vi "From JSON Text (I32).vi"(7 "Default Value":i32, 9 "error in":errorcluster, 10 "Offset":i32, 11 "JSON":string) -> (1 "error out":errorcluster, 3 "Value":i32)   [LabVIEW 2021, in "json.facade.lvlib"]
doc: "Convert JSON to the LabVIEW Data Type entered."
uses:
  jsontext/LVClass Serializer/JSONtext LVClass Serializer.lvclass
  json.facade.lvlib
  jsontext/JSONtext.lvlib
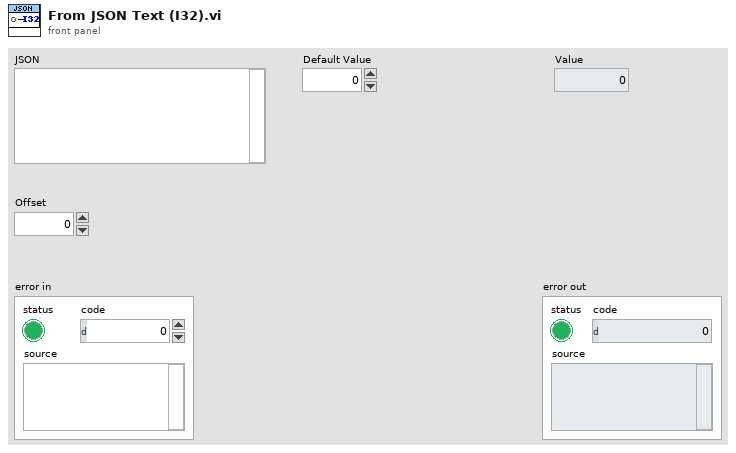
[diagram p1: front panel]
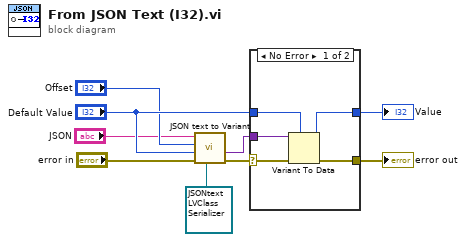
[diagram p0: block diagram]
diagram:
  n1 = call "JSON text to Variant.vi"("LVClass Serializer"=refnum<class "JSONtext LVClass Serializer.lvclass"> refnum, "error in (no error)"="error in", "Data Type"="Default Value", "Offset"="Offset", "JSON"="JSON") -> ("error out"=w2:errorcluster, "Variant out"=w3:variant)  [unwired: 5 in]
  n2 = case shown="No Error" w2 {
    selector: w2 -> [w14 w15]
    tunnel: "Default Value" -> [w12 w16]
    tunnel: [w10 w16] -> w7
    tunnel: w3 -> [w13 _]
    tunnel: [w11 w15] -> w1
    frame No Error {
      n3 = Variant To Data(error in=w14, type=w12, Variant=w13) -> (data=w10:i32, error out=w11:errorcluster)
    }
    frame Error {
    }
  }
  "Value" <- w7
  "error out" <- w1
